vi "Motion Control.vi"() -> ()   [LabVIEW 2014]
uses:
  <vilib>/Utility/miscctls.llb/LVMouseTypeDef.ctl
panel:
  out "Mouse":T1
  in  "stop":bool
  out "2D Picture":picture
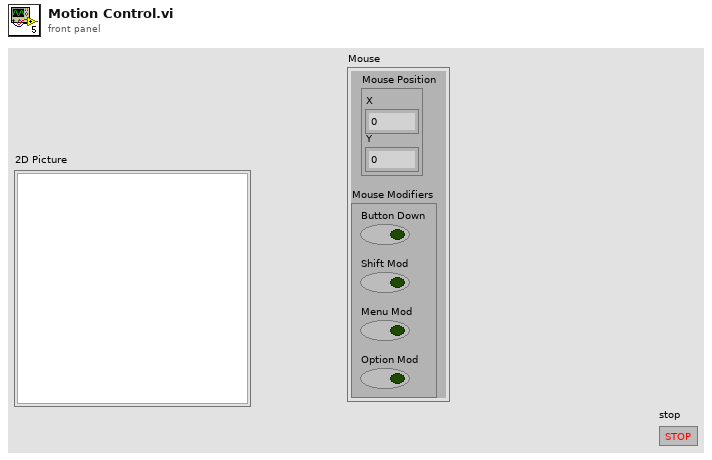
[diagram p1: front panel]
types:
  T1 = typedef "LVMouseTypeDef.ctl" = cluster{"Mouse Position":cluster{"X":i32, "Y":i32}, "Mouse Modifiers":cluster{"Button Down":bool, "Shift Mod":bool, "Menu Mod":bool, "Option Mod":bool}}
  T2 = typedef "LVBoundsTypeDef.ctl" = cluster{"Width":u32, "Height":u32}
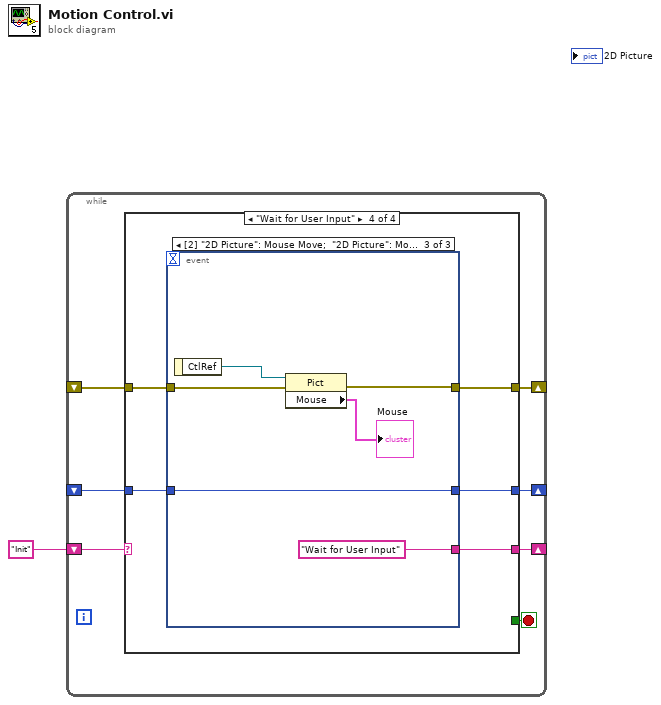
[diagram p0: block diagram]
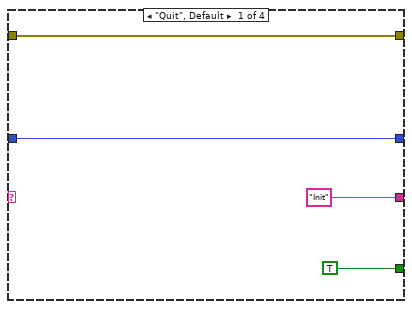
[diagram p2: hidden frame]
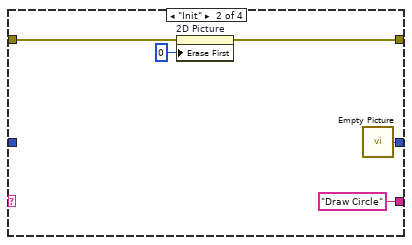
[diagram p3: hidden frame]
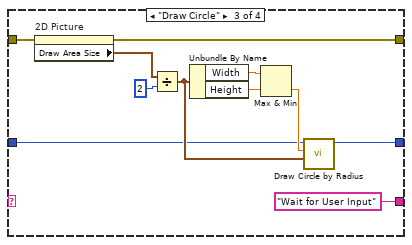
[diagram p4: hidden frame]
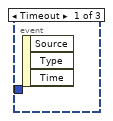
[diagram p5: hidden frame]
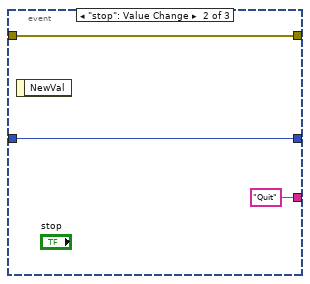
[diagram p6: hidden frame]
diagram:
  n1 = while {
    shift-right: [w6] -> _
    shift-left: "Init" -> [w8]
    shift-right: [w5] -> _
    shift-left: _ -> [w4]
    shift-right: [w3] -> _
    shift-left: _ -> [w2]
    stop <- w7 stop-if-true
    n2 = case shown="\"Wait for User Input\"" w8 {
      tunnel: [TRUE _ _ _] -> w7
      tunnel: ["Init" "Draw Circle" "Wait for User Input" w33] -> w6
      tunnel: [w10 w16 w21 w32] -> w5
      tunnel: w4 -> [w10 w17 w20 w31]
      tunnel: [w9 w15 w19 w30] -> w3
      tunnel: w2 -> [w9 _ w18 w29]
      frame "Quit", Default {
      }
      frame "Init" {
        n3 = property on="2D Picture" class="Pict"(error in=w17, "Erase First"=u8 0) -> (error out=w16:errorcluster)  [unwired: 1 in, 1 out]
        n4 = call "Empty Picture"() -> ("empty picture"=w15:picture)
      }
      frame "Draw Circle" {
        n5 = property on="2D Picture" class="Pict"(error in=w20) -> (error out=w21:errorcluster, "Draw Area Size"=w22:T2)  [unwired: 1 in, 1 out]
        n6 = Divide(x=w22, y=2) -> (x/y=w24:cluster{"Width":dbl, "Height":dbl})
        n7 = Unbundle By Name(w24) -> ("Width"=w25:dbl, "Height"=w26:dbl)
        n8 = Max & Min(x=w25, y=w26) -> (min(x,y)=w27:dbl)  [unwired: 1 out]
        n9 = call <vilib>:"Draw Circle by Radius.vi"("pixel center"=w24, "radius"=w27, "picture"=w18) -> ("new picture"=w19:picture)  [unwired: 8 in]
      }
      frame "Wait for User Input" {
        n10 = event shown="[2] \"2D Picture\": Mouse Move;  \"2D Picture\": Mouse Down;  \"2D Picture\": Mouse Up" {
          selector: _ -> [_ _ _]
          dyn-events: _ -> [_ _ _]
          timeout: _ -> [_ _ _]
          tunnel: [_ "Quit" "Wait for User Input"] -> w33
          tunnel: [_ w35 w40] -> w32
          tunnel: w31 -> [_ w35 w42]
          tunnel: [_ w34 w37] -> w30
          tunnel: w29 -> [_ w34 w37]
          event Timeout {
            n11 = event-data() -> ()  [unwired: 1 in, 3 out]
          }
          event "stop": Value Change {
            n12 = event-data() -> ()  [unwired: 1 in, 1 out]
          }
          event "2D Picture": Mouse Move; "2D Picture": Mouse Down; "2D Picture": Mouse Up {
            n13 = event-data() -> ("CtlRef"=w41:refnum<vi>)  [unwired: 1 in]
            n14 = property class="Pict"(reference=w41, error in=w42) -> (error out=w40:errorcluster, "Mouse"=→"Mouse":T1)  [unwired: 1 out]
          }
        }
      }
    }
  }
